vi "Clear Error.vi"(8 "error in (no error)":errorcluster, 11 "Driver in":refnum<class "Driver.lvclass">) -> (0 "error out":errorcluster, 3 "Driver out":refnum<class "Driver.lvclass">)   [LabVIEW 2023, in "Driver.lvlib" / "Driver.lvclass"]
uses:
  Driver.lvclass
  Driver.lvclass/Driver.ctl
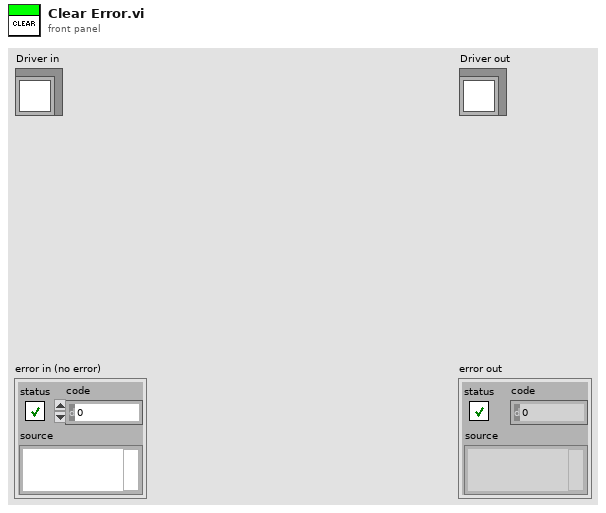
[diagram p1: front panel]
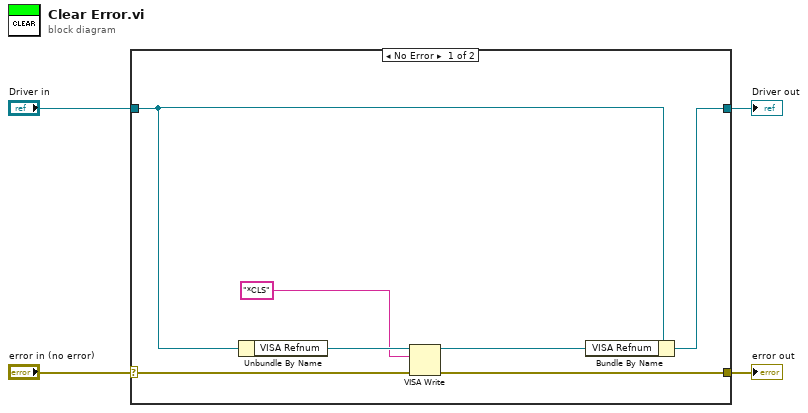
[diagram p0: block diagram]
diagram:
  n1 = case shown="No Error" "error in (no error)" {
    selector: "error in (no error)" -> [w9 w13]
    tunnel: [w8 w13] -> w3
    tunnel: [w6 w12] -> w1
    tunnel: "Driver in" -> [w7 w12]
    frame No Error {
      n2 = Unbundle By Name(w7) -> ("VISA Refnum"=w11:refnum<visa-resource-name>)
      n3 = VISA Write(VISA resource name=w11, write buffer="*CLS", error in (no error)=w9) -> (VISA resource name out=w5:refnum<visa-resource-name>, error out=w8:errorcluster)  [unwired: 1 out]
      n4 = Bundle By Name(cluster=w7, "VISA Refnum"=w5) -> (w6:refnum<class "Driver.lvclass">)
    }
    frame Error {
    }
  }
  "error out" <- w3
  "Driver out" <- w1
